vi "Sync.vi"(8 "error in (no error)":errorcluster, 11 "MQTT-Client in":refnum<class "MQTT-Client.lvclass">) -> (0 "error out":errorcluster, 3 "MQTT-Client out":refnum<class "MQTT-Client.lvclass">)   [LabVIEW 2023, in "MQTT-Client.lvlib" / "MQTT-Client.lvclass"]
uses:
  MQTT-Client.lvclass
  MQTT-Client.lvclass/MQTT-Client.ctl
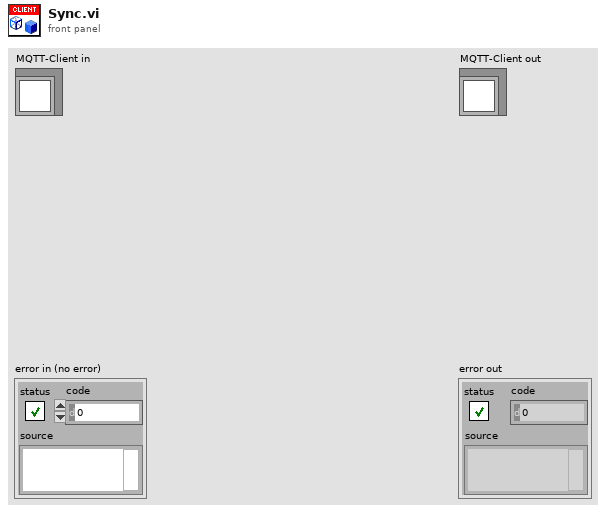
[diagram p1: front panel]
types:
  T1 = typedef "MQTT-Client.lvlib/MQTT-Client.lvclass/Config.ctl" = cluster{"scheduling":i32, "payload":string}
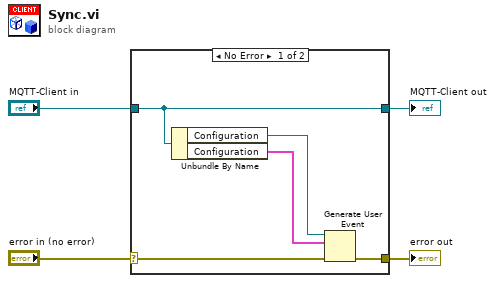
[diagram p0: block diagram]
diagram:
  n1 = case shown="No Error" "error in (no error)" {
    selector: "error in (no error)" -> [w9 w11]
    tunnel: [w8 w11] -> w3
    tunnel: [w7 w10] -> w1
    tunnel: "MQTT-Client in" -> [w7 w10]
    frame No Error {
      n2 = Unbundle By Name(w7) -> ("Configuration"=w6:refnum<user-event>, "Configuration"=w5:T1)
      n3 = Generate User Event(user event=w6, event data cluster=w5, error in=w9) -> (error out=w8:errorcluster)  [unwired: 1 in, 1 out]
    }
    frame Error {
    }
  }
  "error out" <- w3
  "MQTT-Client out" <- w1
